vi "AssertsEqual.vi"(11 "error in (no error)":errorcluster) -> (15 "error out":errorcluster)   [LabVIEW 2016, in "DronaTest.lvlib"]
uses:
  DronaTest.lvlib
  APIs/Assert/AssertControlValue/Equal.vi
  APIs/Stimulus/ControlValue/ValueSignalLatchBooleanString.vi
  <vilib>/addons/_JKI Toolkits/Caraya/classes/Assert/Assert Not Error.vi
  <vilib>/addons/_JKI Toolkits/Caraya/classes/Assert/Assert Error.vi
  <vilib>/addons/_JKI Toolkits/Caraya/classes/Test/Test.lvclass
  Drona.lvlib
  <vilib>/addons/_JKI Toolkits/Caraya/classes/Assert/Assert.lvclass
  APIs/Assert/AssertControlValue/AssertControlValue.lvlib
  APIs/Stimulus/ControlValue/ControlValue.lvlib
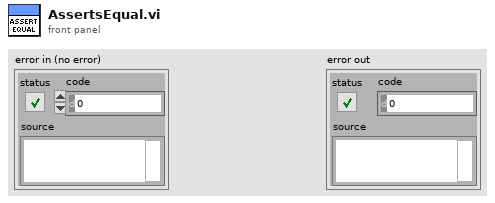
[diagram p1: front panel]
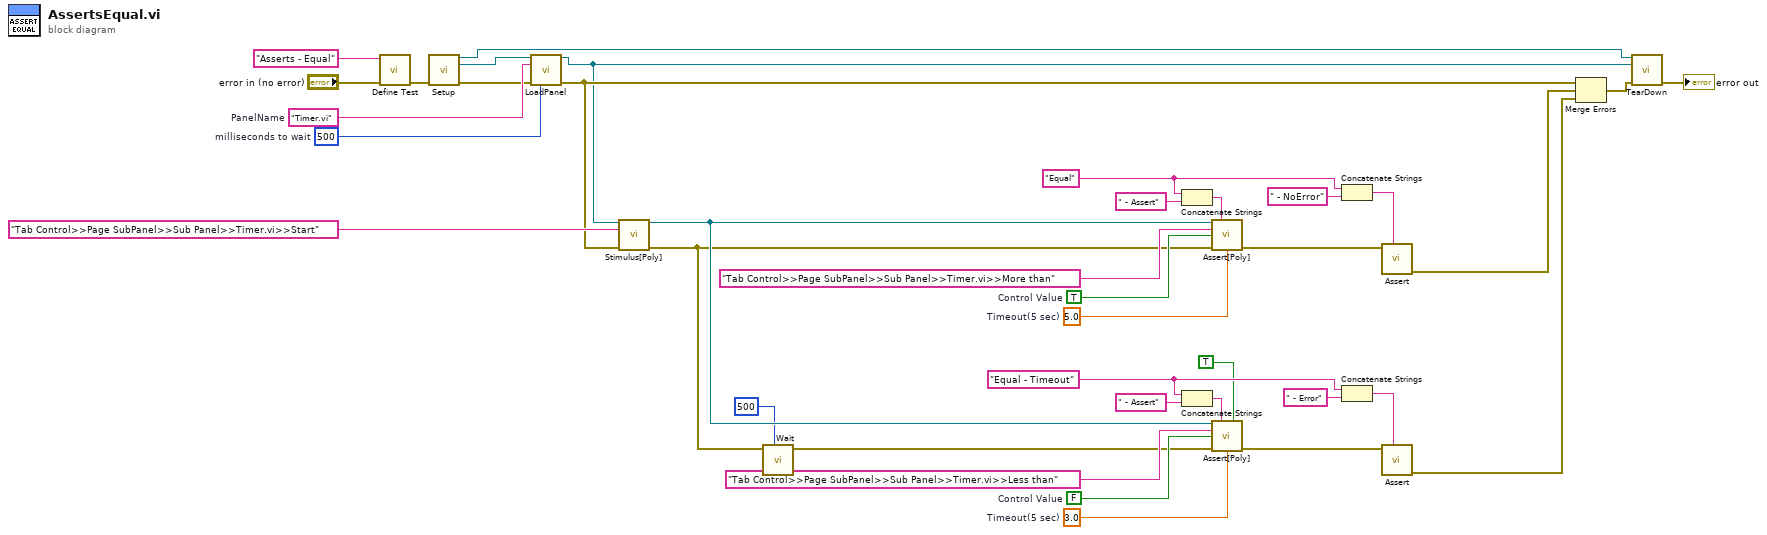
[diagram p0: block diagram]
diagram:
  w9 = u32 500  # milliseconds to wait
  w10 = "Timer.vi"  # PanelName
  w35 = FALSE  # Control Value
  w25 = 3.0  # Timeout(5 sec)
  w24 = "Equal - Timeout" ("string")
  w26 = 5.0  # Timeout(5 sec)
  w27 = TRUE  # Control Value
  w28 = "Equal" ("string")
  n1 = call <vilib>:"Define Test.vi"("error in (no error)"="error in (no error)", "Label (VI Title)"="Asserts - Equal") -> ("error out"=w6:errorcluster)  [unwired: 9 in]
  n2 = call "Setup.vi"("error in (no error)"=w6) -> ("Application Ref"=w2:refnum<vi>, "VI out"=w7:refnum<vi>, "error out"=w8:errorcluster)  [unwired: 12 in]
  n3 = call "LoadPanel.vi"("VI in"=w7, "Panel Name"=w10, "error in (no error)"=w8, "milliseconds to wait"=w9) -> ("VI out"=w1:refnum<vi>, "error out"=w5:errorcluster)  [unwired: 10 in]
  n4 = call-poly "Stimulus[Poly].vi"("VI Reference In"=w1, "Control Path"="Tab Control>>Page SubPanel>>Sub Panel>>Timer.vi>>Start", "error in"=w5) -> ("VI Reference Out"=w16:refnum<vi>, "error out"=w13:errorcluster)  [unwired: 11 in]
  n5 = call "Wait.vi"("milliseconds to wait"=u32 500, "error in (no error)"=w13) -> ("error out"=w12:errorcluster)  [unwired: 9 in]
  n6 = Concatenate Strings(w28, " - Assert" ("string")) -> (w30:string)
  n7 = Concatenate Strings(w24, " - Assert" ("string")) -> (w22:string)
  n8 = call-poly "Assert[Poly].vi"("VI Reference In"=w16, "Test Label"=w30, "Control Path"="Tab Control>>Page SubPanel>>Sub Panel>>Timer.vi>>More than", "Control Value"=w27, "Error In"=w13, "Timeout(5 sec)"=w26) -> ("Error Out"=w31:errorcluster)  [unwired: 8 in, 1 out]
  n9 = call-poly "Assert[Poly].vi"("VI Reference In"=w16, "Test Label"=w22, "Assert Only? (F)"=TRUE, "Control Path"="Tab Control>>Page SubPanel>>Sub Panel>>Timer.vi>>Less than", "Control Value"=w35, "Error In"=w12, "Timeout(5 sec)"=w25) -> ("Error Out"=w21:errorcluster)  [unwired: 7 in, 1 out]
  n10 = Concatenate Strings(w28, " - NoError" ("string")) -> (w29:string)
  n11 = Concatenate Strings(w24, " - Error" ("string")) -> (w23:string)
  n12 = call-poly <vilib>:"Assert.vi"("Label"=w29, "Not Error?"=w31) -> ("error out"=w15:errorcluster)  [unwired: 9 in]
  n13 = call-poly <vilib>:"Assert.vi"("Label"=w23, "Error?"=w21) -> ("error out"=w14:errorcluster)  [unwired: 9 in]
  n14 = Merge Errors(w5, w15, w14) -> (w4:errorcluster)
  n15 = call "TearDown.vi"("Application Ref"=w2, "VI in"=w1, "error in (no error)"=w4) -> ("error out"=→"error out":errorcluster)  [unwired: 12 in]
